vi "Render.vi"(8 "error in (no error)":errorcluster, 10 "String in":string, 11 "Footnote in":refnum<class "Footnote.lvclass">) -> (0 "error out":errorcluster, 2 "String out":string, 3 "Footnote out":refnum<class "Footnote.lvclass">)   [LabVIEW 2021, in "LvMarkdown.lvlib" / "Footnote.lvclass"]
uses:
  Footnote.lvclass
  C:/GitHub/LvMarkdown/src/LvMarkdown/Markdown.lvclass
  Footnote.lvclass/Footnote.ctl
  GetFootnoteReference.vi
  FootnoteReference/FootnoteReference.lvclass
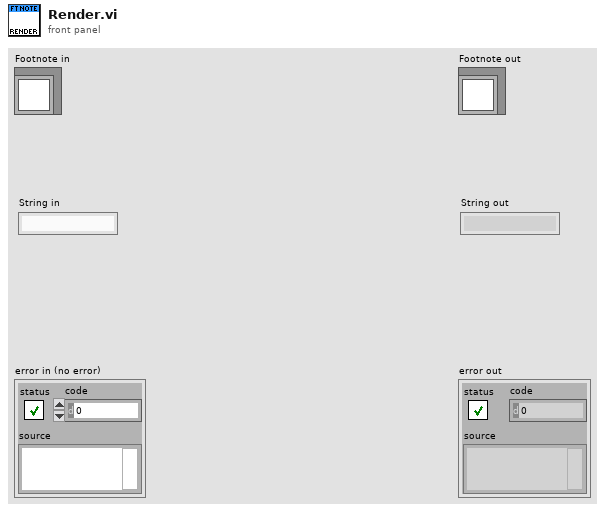
[diagram p1: front panel]
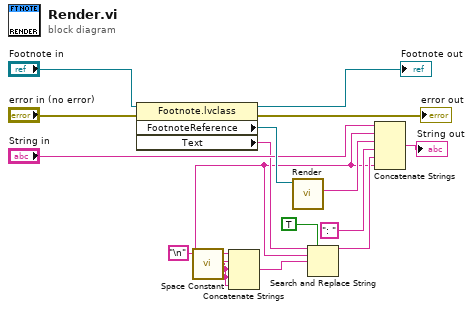
[diagram p0: block diagram]
diagram:
  w2 = "\n"
  n1 = property class="Footnote.lvclass"(reference="Footnote in", error in="error in (no error)") -> (reference out=→"Footnote out":refnum<class "Footnote.lvclass">, error out=→"error out":errorcluster, "FootnoteReference"=w11:refnum<class "FootnoteReference.lvclass">, "Text"=w6:string)
  n2 = call <vilib>:"Space Constant.vi"() -> ("String"=w1:string)
  n3 = Concatenate Strings(w2, w1, w1, w1, w1) -> (w5:string)
  n4 = call-dynamic "Render.vi"("Footnote in"=w11) -> ("String out"=w8:string)  [unwired: 8 in, 2 out]
  n5 = Search and Replace String(replace all?=TRUE ("replace all? (F)"), input string=w6, search string=w2, replace string=w5) -> (result string=w3:string)  [unwired: 4 in, 3 out]
  n6 = Concatenate Strings("String in", w2, w8, ": " ("string"), w3, w2) -> (→"String out":string)
